vi "Sigma_Home.vi"(7 "Axis (1)":string="1", 8 "error in (no error)":errorcluster, 11 "VISA resource name":refnum<visa-resource-name>) -> (0 "error out":errorcluster, 3 "VISA resource name out":refnum<visa-resource-name>)   [LabVIEW 2018]
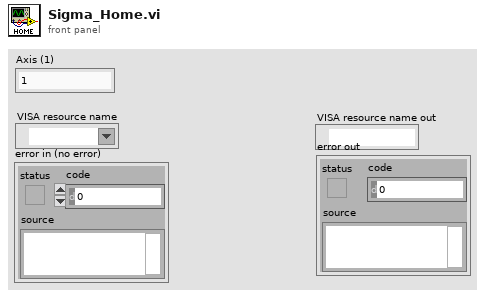
[diagram p1: front panel]
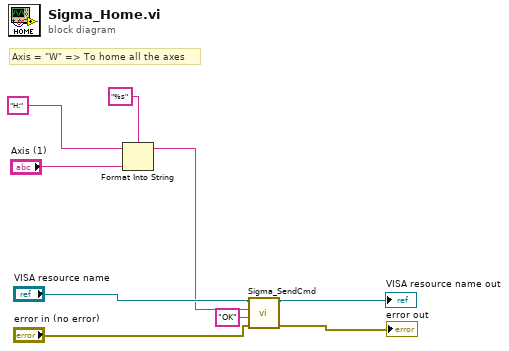
[diagram p0: block diagram]
diagram:
  # "Axis = \"W\" => To home all the axes"
  n1 = Format Into String(format string="%s", initial string="H:" ("string"), "Axis (1)") -> (resulting string=w2:string)  [unwired: 1 in, 1 out]
  n2 = call "Sigma_SendCmd.vi"("error in (no error)"="error in (no error)", "String to Receive"="OK", "String to Send"=w2, "VISA resource name"="VISA resource name") -> ("error out"=→"error out":errorcluster, "VISA resource name out"=→"VISA resource name out":refnum<visa-resource-name>)  [unwired: 4 in, 2 out]
